vi "Log Temp.vi"(8 "error in (no error)":errorcluster, 11 "Temperature Controller in":refnum<class "Temperature Controller.lvclass">) -> (0 "error out":errorcluster, 3 "Temperature Controller out":refnum<class "Temperature Controller.lvclass">)   [LabVIEW 2009, in "Temperature Controller.lvclass"]
uses:
  Temperature Controller.lvclass
  Global/File Locations.vi
  File IO/File IO.lvclass
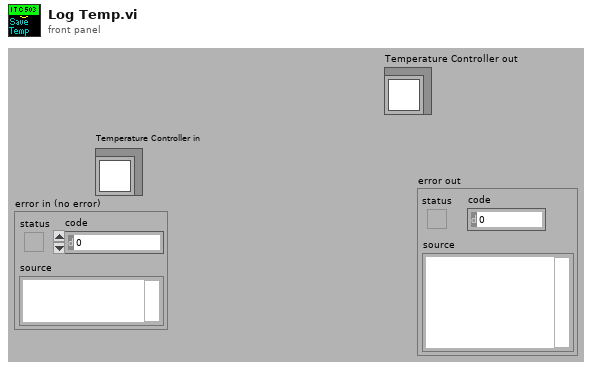
[diagram p1: front panel]
types:
  T1 = enum16{"open", "open or create", "create or replace", "create", "open (read only)"}
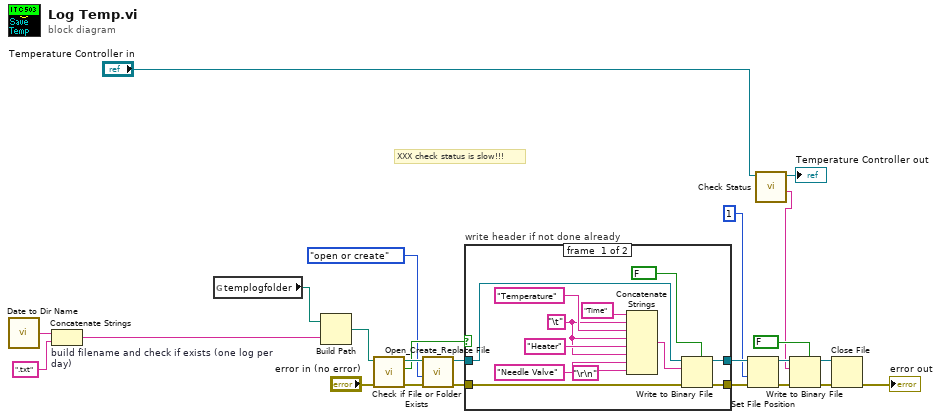
[diagram p0: block diagram]
diagram:
  # "XXX check status is slow!!!"
  n1 = call "Date to Dir Name.vi"() -> ("Dir Name"=w24:string)
  n2 = Concatenate Strings "build filename and check if exists (one log per day)"(w24, ".txt") -> (w7:string)
  n3 = global read "File Locations.vi" "templogfolder"() -> (w6:path)
  n4 = Build Path(base path=w6, name or relative path=w7) -> (appended path=w5:path)
  n5 = call <vilib>:"Check if File or Folder Exists.vi"("error in (no error)"="error in (no error)", "path"=w5) -> ("error out"=w12:errorcluster, "file or folder exists?"=w21:bool, "dup path"=w22:path)  [unwired: 7 out]
  n6 = call <vilib>:"Open_Create_Replace File.vi"("error in (no error)"=w12, "function (open:0)"=T1."open or create", "file path"=w22) -> ("error out"=w19:errorcluster, "refnum"=w20:refnum<file>)  [unwired: 3 in, 4 out]
  n7 = case "write header if not done already" shown="False" w21 {
    tunnel: w20 -> [w36 w38]
    tunnel: w19 -> [w35 w37]
    tunnel: [w34 w37] -> w17
    tunnel: [w26 w38] -> w18
    frame #0 {
      w29 = "\t"
      n8 = Concatenate Strings("Time", w29, "Temperature", w29, "Heater", w29, "Needle Valve", "\r\n") -> (w28:string)
      n9 = Write to Binary File(file (use dialog)=w36, data=w28, error in=w35, 5:FALSE ("prepend array or string size? (T)")) -> (refnum out=w26:refnum<file>, error out=w34:errorcluster)  [unwired: 3 out]
    }
    frame #1 {
    }
  }
  n10 = Set File Position(refnum=w18, from (0:start)=1, error in=w17) -> (refnum out=w11:refnum<file>, error out=w10:errorcluster)  [unwired: 1 out]
  n11 = call-dynamic "Check Status.vi"("Temperature Controller in"="Temperature Controller in") -> ("Status"=w3:string, "Temperature Controller out"=→"Temperature Controller out":refnum<class "Temperature Controller.lvclass">)  [unwired: 7 in, 2 out]
  n12 = Write to Binary File(file (use dialog)=w11, data=w3, error in=w10, 5:FALSE ("prepend array or string size? (T)")) -> (refnum out=w16:refnum<file>, error out=w14:errorcluster)  [unwired: 3 out]
  n13 = Close File(refnum=w16, error in=w14) -> (error out=→"error out":errorcluster)  [unwired: 1 out]
